vi "subvi_move_to_set_angle.vi"(8 "file (use dialog)":path, 10 "Current Angles":cluster{"Analyser 1":i32, "Analyser 2":i32}, 11 "Analyser Set Angles":cluster{"Analyser 1":i32, "Analyser 2":i32}) -> (1 "Crenelation \nInterrupts":bool[](array[boolean]) caption="Crenelation Indicators", 2 "New Current Angles":cluster{"Analyser 1":i32, "Analyser 2":i32}, 3 "Analysers Moving?":T1, 4 "A2 Crenelation Interrupt State":i16(graph), 6 "A1 Crenelation Interrupt State":i16(graph))   [LabVIEW 2014]
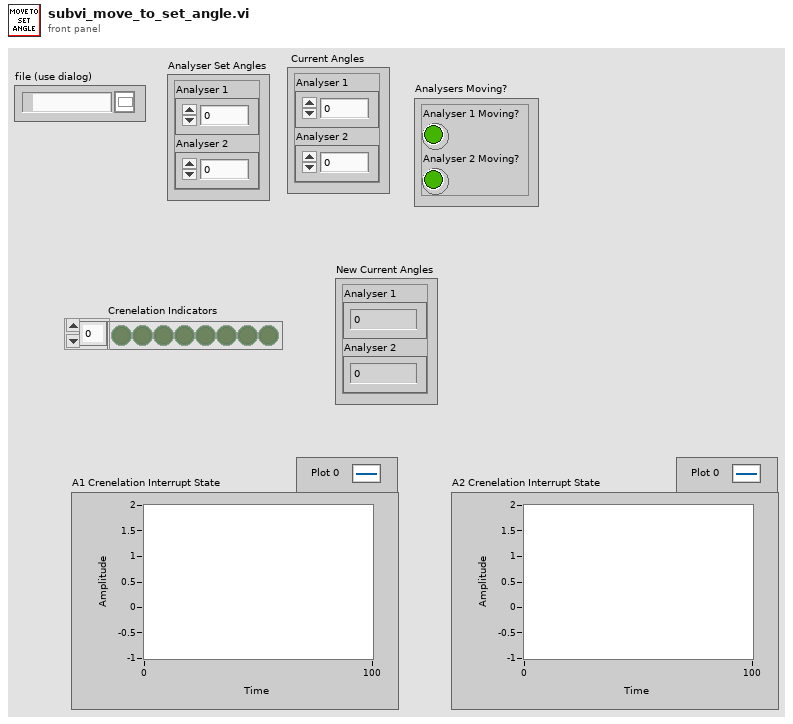
[diagram p1: front panel]
types:
  T1 = cluster{"Analyser 1 Moving?":bool, "Analyser 2 Moving?":bool}
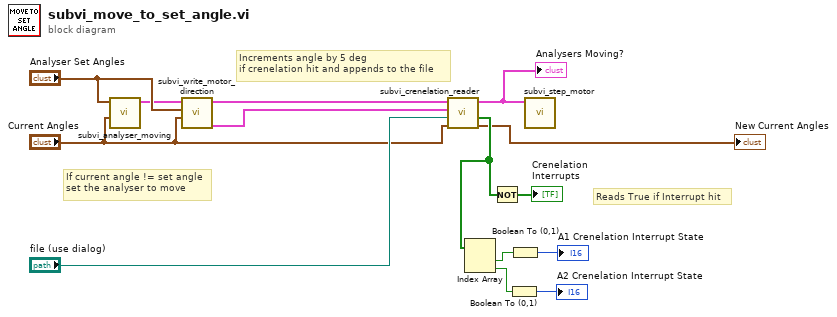
[diagram p0: block diagram]
diagram:
  # "Reads True if Interrupt hit"
  # "Increments angle by 5 deg\nif crenelation hit and appends to the file"
  # "If current angle != set angle\nset the analyser to move"
  n1 = call "subvi_analyser_moving.vi"("Current Angles"="Current Angles", "Set Angles"="Analyser Set Angles") -> ("Analysers Moving?"=w1:T1)  [unwired: 9 in]
  n2 = call "subvi_write_motor_direction.vi"("Current Angles"="Current Angles", "Set Angles"="Analyser Set Angles", "Analysers Moving?"=w1) -> ("Directions"=w5:cluster{"Analyser 1":bool, "Analyser 2":bool}, "Analysers Moving? Output"=w4:T1)  [unwired: 7 in]
  n3 = call "subvi_crenelation_reader.vi"("Current Angles"="Current Angles", "file (use dialog) 2"="file (use dialog)", "Directions"=w5, "Analysers Moving?"=w4) -> ("New Current Angles"=→"New Current Angles":cluster{"Analyser 1":i32, "Analyser 2":i32}, "Crenelation \nInterrupts"=w13:bool[], "Analysers Moving? Output"=w7:T1)  [unwired: 5 in]
  "Analysers Moving?" <- w7
  n4 = Index Array(array=w13) -> (element #1=w10:bool, element #2=w12:bool)  [unwired: 2 in]
  n5 = Not(x=w13) -> (.not. x?=→"Crenelation \nInterrupts":bool[])
  n6 = Boolean To (0,1)(Boolean=w12) -> (0, 1=→"A2 Crenelation Interrupt State":i16)
  n7 = Boolean To (0,1)(Boolean=w10) -> (0, 1=→"A1 Crenelation Interrupt State":i16)
  n8 = call "subvi_step_motor.vi"("Write to Motor?"=w7) -> ()  [unwired: 11 in]
